vi "Waveform_Read Write End Point Index.vi"(6 "Read(f)\nWrite(t)":T1, 8 "Error":errorcluster, 10 "End Point":i32, 11 "Waveform Attributes":variant) -> (0 "Error Out":errorcluster, 1 "Success":bool, 2 "End Point Out":i32, 3 "Waveform Attributes Out":variant)   [LabVIEW 2020]
uses:
  Universal Controls/Read Write Button.ctl
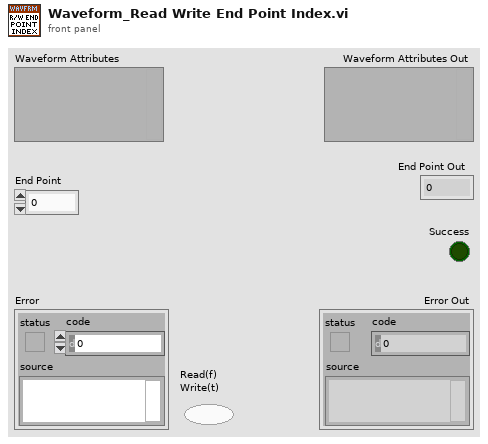
[diagram p1: front panel]
types:
  T1 = typedef "Read Write Button.ctl" = bool
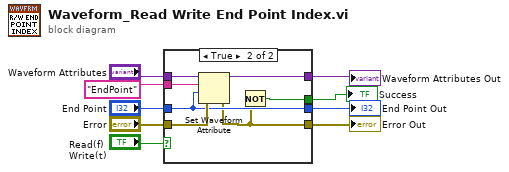
[diagram p0: block diagram]
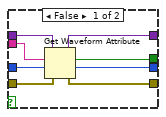
[diagram p2: hidden frame]
diagram:
  n1 = case shown="True" "Read(f)\nWrite(t)" {
    tunnel: [w17 w21] -> w9
    tunnel: "Waveform Attributes" -> [w16 w22]
    tunnel: "End Point" -> [w15 w20]
    tunnel: "EndPoint" ("name") -> [w14 w24]
    tunnel: "Error" -> [w13 w23]
    tunnel: [w12 w19] -> w4
    tunnel: [w11 w20] -> w3
    tunnel: [w10 w18] -> w1
    frame False {
      n2 = Get Waveform Attribute(4:w13, 5:w15, 6:w14, 7:w16) -> (0:w12:errorcluster, 1:w11:i32, 2:w10:bool, 3:w17:variant)
    }
    frame True {
      n3 = Set Waveform Attribute(4:w23, 5:w20, 6:w24, 7:w22) -> (0:w19:errorcluster, 3:w21:variant)  [unwired: 1 out]
      n4 = Not(x=w19) -> (.not. x?=w18:bool)
    }
  }
  "Waveform Attributes Out" <- w9
  "Error Out" <- w4
  "End Point Out" <- w3
  "Success" <- w1
